vi "Maintenance GV.vi"() -> ()   [LabVIEW 2021]
uses:
  support/Controls/All Inputs.ctl
  RT/Controls/DI 1.ctl
  RT/Controls/DI 2.ctl
  RT/Controls/DO 1.ctl
  support/Controls/Index Details.ctl
panel:
  in  "Index Details":T1
  in  "All IO":T2
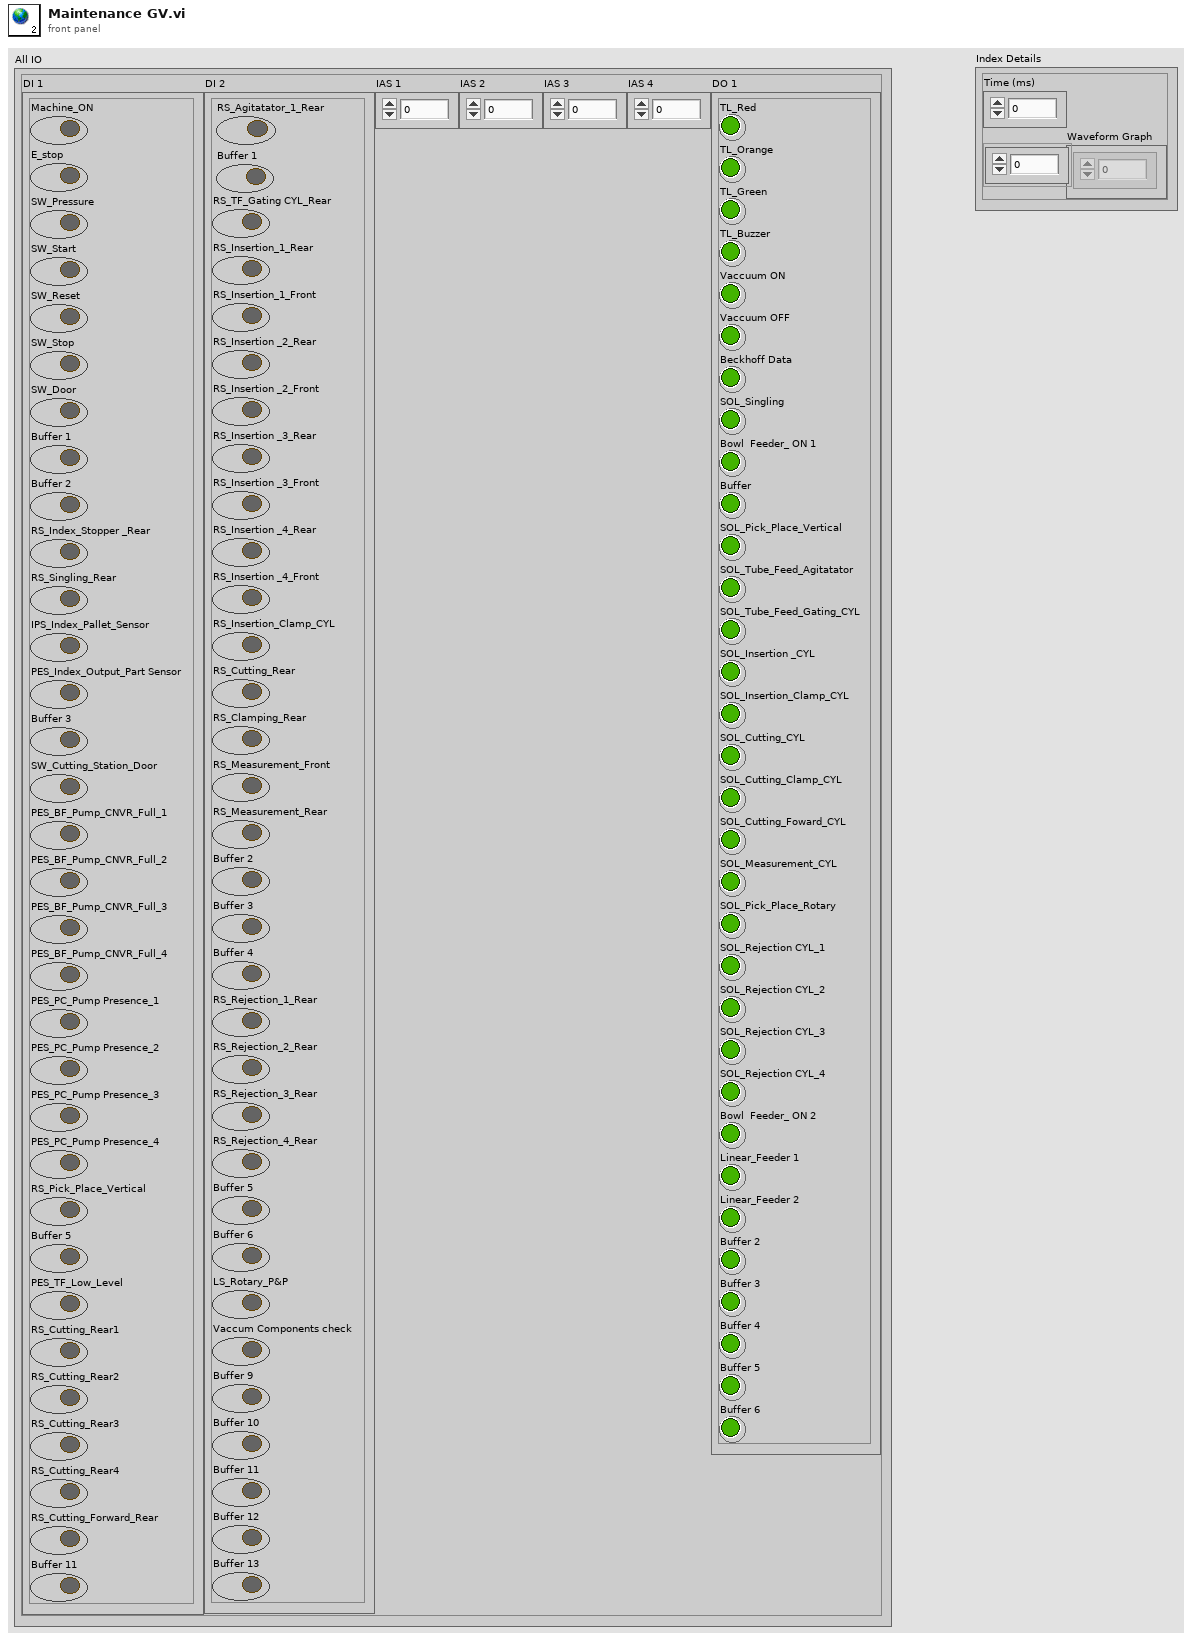
[diagram p1: front panel]
types:
  T1 = typedef "Index Details.ctl" = cluster{"Time (ms)":u32, "Waveform Graph":i16[]}
  T2 = typedef "All Inputs.ctl" = cluster{"DI 1":T3, "DI 2":T4, "IAS 1":dbl, "IAS 2":dbl, "IAS 3":dbl, "IAS 4":dbl, "DO 1":T5}
  T3 = typedef "DI 1.ctl" = cluster{"Machine_ON":bool, "E_stop ":bool, "SW_Pressure":bool, "SW_Start ":bool, "SW_Reset":bool, "SW_Stop":bool, "SW_Door":bool, "Buffer 1":bool, "Buffer 2":bool, "RS_Index_Stopper _Rear":bool, "RS_Singling_Rear":bool, "IPS_Index_Pallet_Sensor":bool, "PES_Index_Output_Part Sensor":bool, "Buffer 3":bool, "SW_Cutting_Station_Door":bool, "PES_BF_Pump_CNVR_Full_1":bool, "PES_BF_Pump_CNVR_Full_2":bool, "PES_BF_Pump_CNVR_Full_3":bool, "PES_BF_Pump_CNVR_Full_4":bool, "PES_PC_Pump Presence_1":bool, "PES_PC_Pump Presence_2":bool, "PES_PC_Pump Presence_3":bool, "PES_PC_Pump Presence_4":bool, "RS_Pick_Place_Vertical":bool, "Buffer 5":bool, "PES_TF_Low_Level":bool, "RS_Cutting_Rear1":bool, "RS_Cutting_Rear2":bool, "RS_Cutting_Rear3":bool, "RS_Cutting_Rear4":bool, "RS_Cutting_Forward_Rear":bool, "Buffer 11":bool}
  T4 = typedef "DI 2.ctl" = cluster{"RS_Agitatator_1_Rear":bool, "Buffer 1 ":bool, "RS_TF_Gating CYL_Rear":bool, "RS_Insertion_1_Rear":bool, "RS_Insertion_1_Front":bool, "RS_Insertion _2_Rear":bool, "RS_Insertion _2_Front":bool, "RS_Insertion _3_Rear":bool, "RS_Insertion _3_Front":bool, "RS_Insertion _4_Rear":bool, "RS_Insertion _4_Front":bool, "RS_Insertion_Clamp_CYL":bool, "RS_Cutting_Rear":bool, "RS_Clamping_Rear":bool, "RS_Measurement_Front":bool, "RS_Measurement_Rear":bool, "Buffer 2":bool, "Buffer 3":bool, "Buffer 4":bool, "RS_Rejection_1_Rear":bool, "RS_Rejection_2_Rear":bool, "RS_Rejection_3_Rear":bool, "RS_Rejection_4_Rear":bool, "Buffer 5":bool, "Buffer 6":bool, "LS_Rotary_P&P":bool, "Vaccum Components check":bool, "Buffer 9":bool, "Buffer 10":bool, "Buffer 11":bool, "Buffer 12":bool, "Buffer 13":bool}
  T5 = typedef "DO 1.ctl" = cluster{"TL_Red":bool, "TL_Orange":bool, "TL_Green":bool, "TL_Buzzer":bool, "Vaccuum ON":bool, "Vaccuum OFF":bool, "Beckhoff Data":bool, "SOL_Singling":bool, "Bowl  Feeder_ ON 1":bool, "Buffer":bool, "SOL_Pick_Place_Vertical":bool, "SOL_Tube_Feed_Agitatator":bool, "SOL_Tube_Feed_Gating_CYL":bool, "SOL_Insertion _CYL":bool, "SOL_Insertion_Clamp_CYL":bool, "SOL_Cutting_CYL":bool, "SOL_Cutting_Clamp_CYL":bool, "SOL_Cutting_Foward_CYL":bool, "SOL_Measurement_CYL":bool, "SOL_Pick_Place_Rotary":bool, "SOL_Rejection CYL_1":bool, "SOL_Rejection CYL_2":bool, "SOL_Rejection CYL_3":bool, "SOL_Rejection CYL_4":bool, "Bowl  Feeder_ ON 2":bool, "Linear_Feeder 1":bool, "Linear_Feeder 2":bool, "Buffer 2":bool, "Buffer 3":bool, "Buffer 4":bool, "Buffer 5":bool, "Buffer 6":bool}
diagram:
